vi "Write Control Refnum Values from Object Items.vi"(6 "Generate Value Change Events?":T1, 7 "$Path or Item Name":string caption="Object $Path or Item Name", 8 "error in (no error)":errorcluster, 9 "Control References":refnum<vi>[](array[refnum]), 10 "Offset":i32, 11 "JSON":string) -> (0 "error out":errorcluster)   [LabVIEW 2021, in "json.facade.lvlib"]
doc: "Write the the Value Property of the input Control References. Control Labels are used to identify item names in the JSON; Controls are writen with the corresponding JSON items. \n\nOptionally, Value (Signalling) may be used, to trigger Value Change Events.\n\nSee Detailed Help on JSON Path expressions supported by JSONtext."
uses:
  json.facade.lvlib
  jsontext/JSONtext.lvlib
  jsontext/LVClass Serializer/JSONtext LVClass Serializer.lvclass
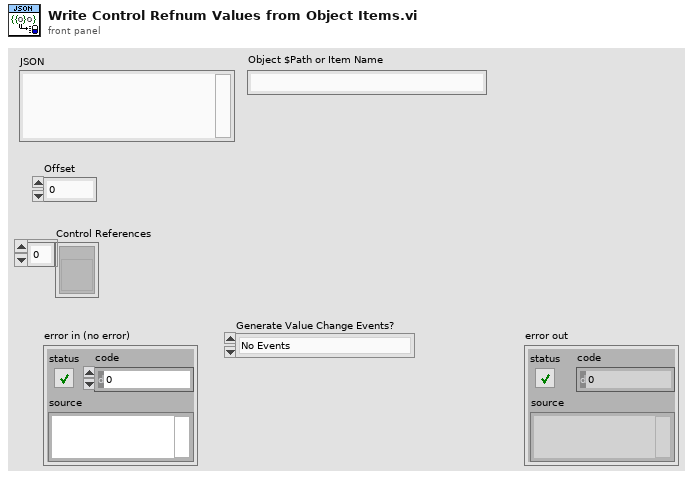
[diagram p1: front panel]
types:
  T1 = typedef "JSONtext.lvlib/Value Change Event Behaviour" = enum16{"No Events", "If found in JSON", "All Controls"}
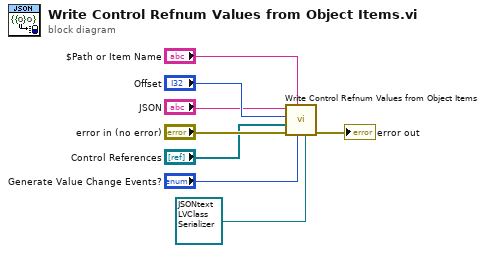
[diagram p0: block diagram]
diagram:
  n1 = call "Write Control Refnum Values from Object Items.vi"("LVClass Serializer"=refnum<class "JSONtext LVClass Serializer.lvclass"> refnum, "Generate Value Change Events?"="Generate Value Change Events?", "$Path or Item Name"="$Path or Item Name", "error in (no error)"="error in (no error)", "Control References"="Control References", "Offset"="Offset", "JSON"="JSON") -> ("error out"=→"error out":errorcluster)  [unwired: 4 in]
